vi "RT Loop - Analyze Acceleration_3.vi"(7 "testing":bool, 8 "error in (no error)":errorcluster, 9 "Acceleration RT FIFO In":T1, 10 "FPGA VI Reference Out":refnum<k20>, 11 "Message Queue":refnum<queue>) -> (1 "Acceleration RT FIFO Out":T1)   [LabVIEW 2017]
doc: "Read and analyze acceleration waveform data from FPGA via DMA FIFO. If the acceleration is over the limit, then send the acceleration waveform data to the Log Data Loop."
uses:
  UI Error Handlers/support/Message Queue/Message Cluster.ctl
  controls/Acceleration RT FIFO Reference.ctl
  Globals/Global - All RT Loop Stop.vi
  Globals/Global - Configuration Options.vi
  <vilib>/Utility/error.llb/Error Cluster From Error Code.vi
  <vilib>/rvi/errors/niLvFpgaAdjustHostInterfaceError.vi
  <vilib>/rvi/interface/nirviMethod/nirviMethod.xnode
  <vilib>/FPGAPlugInAG/Dynamic/niLvFpga_ReadFifo_Dynamic.vi
  <vilib>/rvi/errors/niLvFpgaMergeErrorWithErrorCode.vi
  UI Error Handlers/support/Logging/Logging.lvlib
  UI Error Handlers/support/Message Queue/Message Queue.lvlib
panel:
  out "Array":waveform(dbl)[](array[waveform])
  out "x-y":u32
  out "G1 status.G1 trigger":bool
  out "sta":bool
  out "logical OR":bool
  in  "Data Rate (Hz)":dbl
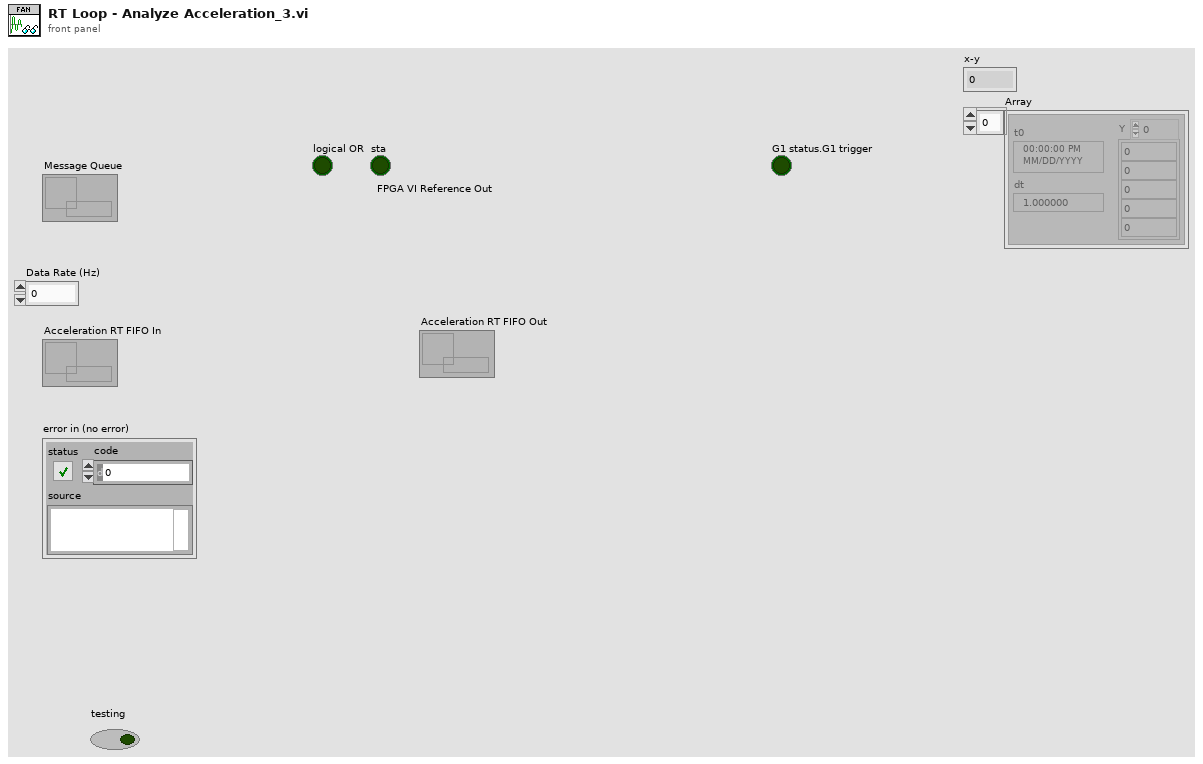
[diagram p1: front panel]
types:
  T1 = typedef "Acceleration RT FIFO Reference.ctl" = refnum<k33>
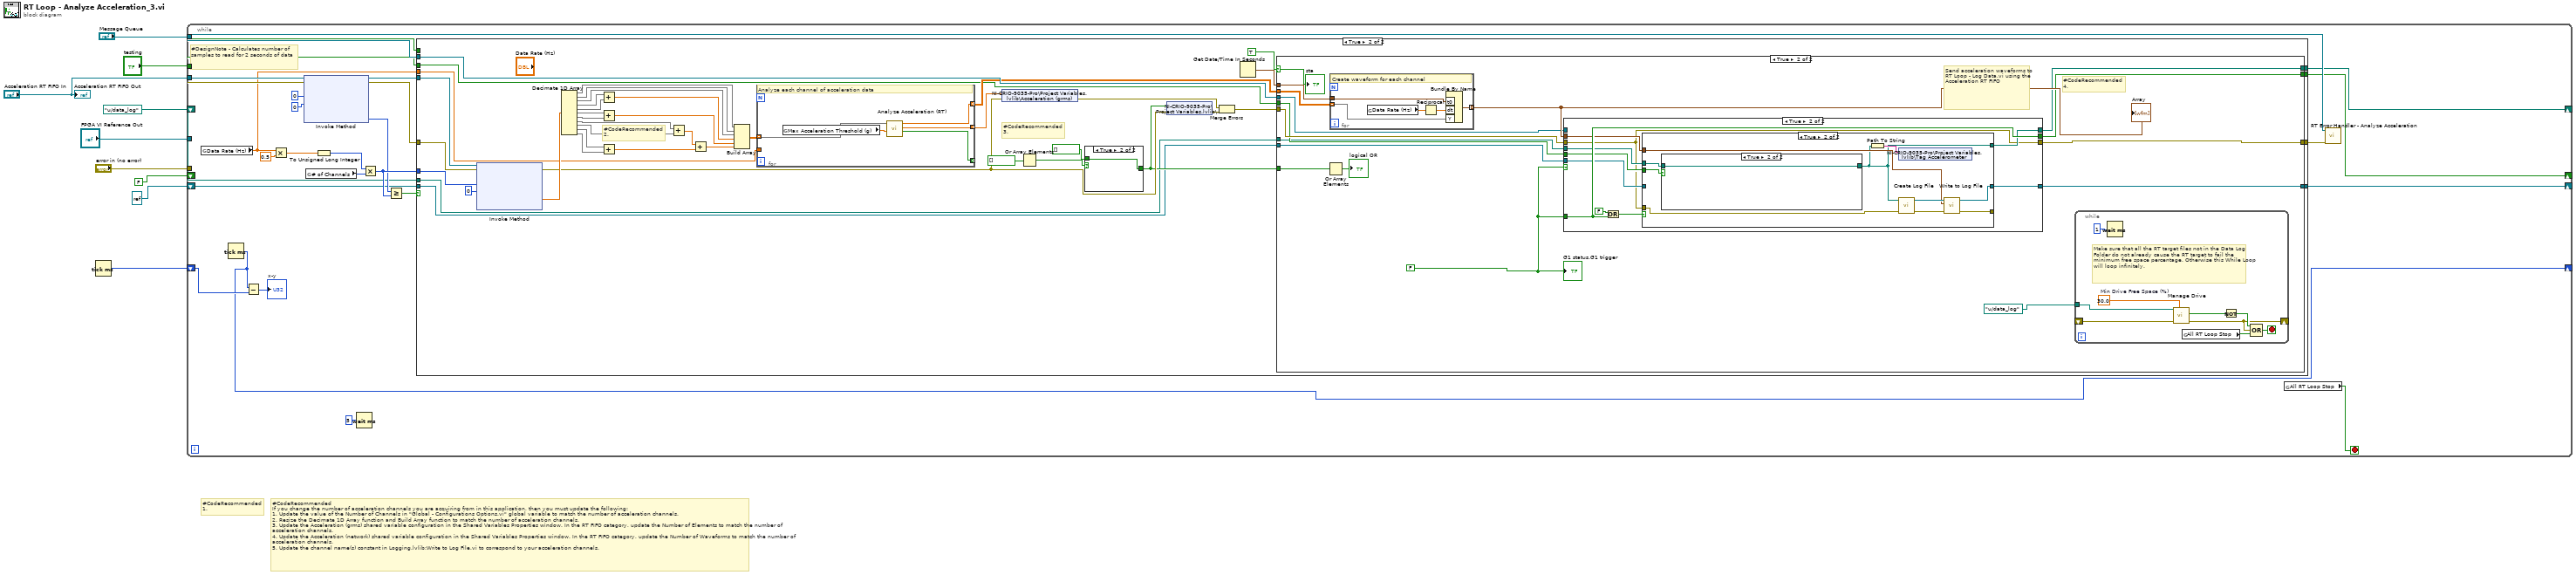
[diagram p0: block diagram]
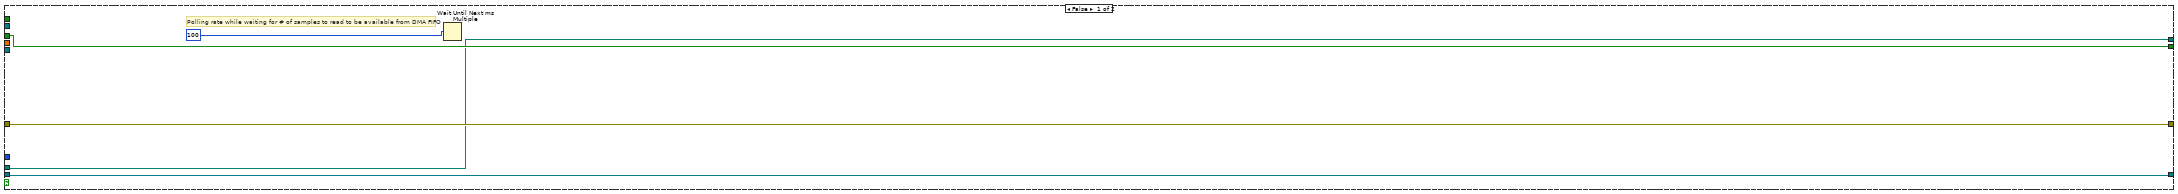
[diagram p2: hidden frame]
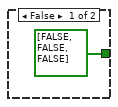
[diagram p3: hidden frame]
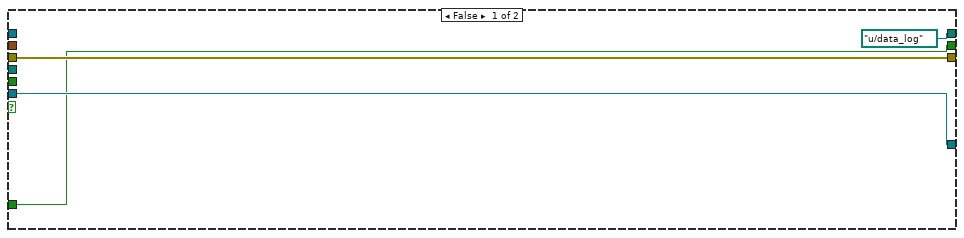
[diagram p5: hidden frame]
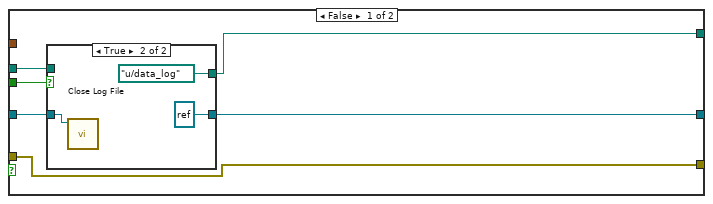
[diagram p6: hidden frame]
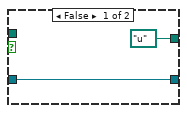
[diagram p7: hidden frame]
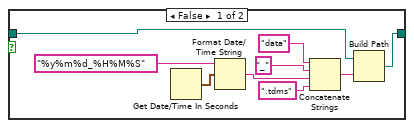
[diagram p8: hidden frame]
diagram:
  # "#CodeRecommended\n1."
  # "#CodeRecommended\nIf you change the number of acceleration channels you are acquiring from in this application, then you must update the following:\n1. Update the value of the Number of Channels in \"Global - Configurations Options.vi\" global variable to match the number of acceleration channels.\n2. Resize the Decimate 1D Array function and Build Array function to match the number of acceleration channels. \n3. Update the Acceleration (grms) shared variable configuration in the Shared Variables Properties window. In the RT FIFO category, update the Number of Elements to match the number of acceleration channels. \n4. Update the Acceleration (network) shared variable configuration in the Shared Variables Properties window. In the RT FIFO category, update the Number of Waveforms to match the number of acceleration channels.\n5. Update the channel name(s) constant in Logging.lvlib:Write to Log File.vi to correspond to your acceleration channels."
  n1 = Tick Count (ms)() -> (millisecond timer value=w1:u32)
  n2 = while {
    tunnel: "FPGA VI Reference Out" -> [w38]
    tunnel: "error in (no error)" -> [w37]
    tunnel: "Message Queue" -> [w30]
    tunnel: "Acceleration RT FIFO In" -> [w28]
    tunnel: "testing" -> [w20]
    shift-right: [w17] -> _
    shift-left: path "u:/data_log" ("AVI Path") -> [w16]
    shift-right: [w19] -> _
    shift-left: FALSE -> [w18]
    shift-right: [w15] -> _
    shift-left: refnum<k34> refnum ("Log File out") -> [w14]
    shift-right: [w12] -> _
    shift-left: w1 -> [w13]
    stop <- w31 stop-if-true
    # "#DesignNote - Calculates number of samples to read for 2 seconds of data"
    n3 = global read "Global - Configuration Options.vi" "Data Rate (Hz)"() -> (w22:dbl)
    n4 = Tick Count (ms)() -> (millisecond timer value=w12:u32)
    n5 = Subtract(x=w12, y=w13) -> (x-y=→"x-y":u32)
    n6 = Multiply(x=w22, y=0.5) -> (x*y=w26:dbl)
    n7 = xnode "Invoke Method"("FPGA VI Reference In"=w38, "error in"=w37, "Number of Elements"=u32 0, "Timeout (ms)"=0) -> ("FPGA VI Reference Out"=w34:refnum<k20>, "error out"=w33:errorcluster, "Elements Remaining"=w21:u32)  [unwired: 1 out]
    n8 = global read "Global - Configuration Options.vi" "# of Channels"() -> (w23:u32)
    n9 = To Unsigned Long Integer(number=w26) -> (unsigned 32bit integer=w25:u32)
    n10 = Wait (ms)(milliseconds to wait=u32 5) -> ()  [unwired: 1 out]
    n11 = Multiply(x=w25, y=w23) -> (x*y=w24:u32)
    n12 = Greater Or Equal?(x=w21, y=w24) -> (x >= y?=w32:bool)
    n13 = case shown="True" w32 {
      tunnel: w34 -> [_ w86]
      tunnel: w33 -> [w43 w85]
      tunnel: [w43 w81] -> w29
      tunnel: w24 -> [_ w84]
      tunnel: w28 -> [_ w80]
      tunnel: w22 -> [_ w76]
      tunnel: w20 -> [_ _]
      tunnel: [w41 w69] -> w19
      tunnel: w18 -> [w41 w68]
      tunnel: [w40 w67] -> w17
      tunnel: w16 -> [w40 w66]
      tunnel: [w39 w65] -> w15
      tunnel: w14 -> [w39 w64]
      frame False {
        # "Polling rate while waiting for # of samples to read to be available from DMA FIFO"
        n14 = Wait Until Next ms Multiple(millisecond multiple=u32 100) -> ()  [unwired: 1 out]
      }
      frame True {
        # "#CodeRecommended\n3."
        # "#CodeRecommended\n2."
        n15 = xnode "Invoke Method"("FPGA VI Reference In"=w86, "error in"=w85, "Number of Elements"=w84, "Timeout (ms)"=0) -> ("error out"=w75:errorcluster, "Data"=w79:sgl[])  [unwired: 2 out]
        n16 = Decimate 1D Array(w79) -> (w61:sgl[], w60:sgl[], w59:sgl[], w58:sgl[], w57:sgl[], w55:sgl[], w54:sgl[], w53:sgl[], w52:sgl[], w51:sgl[], w50:sgl[])
        n17 = Add(x=w58, y=w57) -> (x+y=w56:sgl[])
        n18 = Add(x=w55, y=w54) -> (x+y=w46:sgl[])
        n19 = Add(x=w51, y=w50) -> (x+y=w48:sgl[])
        n20 = Add(x=w53, y=w52) -> (x+y=w49:sgl[])
        n21 = Add(x=w49, y=w48) -> (x+y=w47:sgl[])
        n22 = Build Array(w61, w60, w59, w56, w46, w47) -> (w62:sgl[][])
        n23 = for {
          tunnel: [w93] -> _ mode=indexing
          tunnel: [w92] -> w78 mode=indexing
          tunnel: [w91] -> w77 mode=indexing
          tunnel: w76 -> [_]
          tunnel: w62 -> [w89] mode=indexing
          # "Analyze each channel of acceleration data"
          n24 = global read "Global - Configuration Options.vi" "Max Acceleration Threshold (g)"() -> (w90:sgl)
          n25 = call "Analyze Acceleration (RT).vi"("Max Instantaneous Acceleration (g)"=w90, "Acceleration Waveform (SGL)"=w89) -> ("Over Limit?"=w93:bool, "Acceleration (grms)"=w91:dbl, "Acceleration Waveform (DBL)"=w92:dbl[])  [unwired: 7 in]
        }
        n26 = shared-variable "NI-CRIO-9035-Pro\\Project Variables.lvlib\\Acceleration (grms)"(w77, error in=w75) -> (error out=w73:errorcluster)
        n27 = Or Array Elements(Boolean array=bool[] []) -> (logical OR=w71:bool)
        n28 = case shown="True" w71 {
          tunnel: bool[] [] -> [_ w88]
          tunnel: [bool[] [FALSE, FALSE, FALSE] ("Chatter?") w88] -> w70
          frame False {
          }
          frame True {
          }
        }
        n29 = shared-variable "NI-CRIO-9035-Pro\\Project Variables.lvlib\\Chatter?"(w70, error in=w75) -> (error out=w74:errorcluster)
        n30 = Merge Errors(w73, w74) -> (w72:errorcluster)
        n31 = Get Date/Time In Seconds() -> (seconds since 1Jan1904=w82:timestamp)
        n32 = case shown="True" TRUE {
          selector: TRUE -> [_ w107]
          tunnel: w82 -> [_ w114]
          tunnel: w72 -> [w97 w113]
          tunnel: [w97 w98] -> w81
          tunnel: w80 -> [_ w111]
          tunnel: w78 -> [_ w110]
          tunnel: w70 -> [_ w108]
          tunnel: [w96 w106] -> w69
          tunnel: w68 -> [w96 w105]
          tunnel: [w95 w104] -> w67
          tunnel: w66 -> [w95 w101]
          tunnel: [w94 w103] -> w65
          tunnel: w64 -> [w94 w102]
          frame False {
          }
          frame True {
            w99 = FALSE
            # "#CodeRecommended\n4."
            # "Send acceleration waveforms to RT Loop - Log Data.vi using the Acceleration RT FIFO"
            n33 = Or Array Elements(Boolean array=w108) -> (logical OR=→"logical OR":bool)
            n34 = for {
              tunnel: w110 -> [w173] mode=indexing
              tunnel: w114 -> [w172]
              tunnel: [w170] -> w112 mode=indexing
              # "Create waveform for each channel"
              n35 = global read "Global - Configuration Options.vi" "Data Rate (Hz)"() -> (w169:dbl)
              n36 = Reciprocal(x=w169) -> (1/x=w171:dbl)
              n37 = Bundle By Name("t0"=w172, "dt"=w171, "Y"=w173) -> (w170:waveform(dbl))  [unwired: 1 in]
            }
            "Array" <- w112
            n38 = case shown="True" w99 {
              tunnel: w113 -> [w127 w128]
              tunnel: w112 -> [_ w129]
              tunnel: w111 -> [_ _]
              tunnel: w99 -> [w125 w135]
              tunnel: [w125 w135] -> w106
              tunnel: w105 -> [_ w134]
              tunnel: [path "u:/data_log" ("AVI Path") w133] -> w104
              tunnel: w101 -> [_ w132]
              tunnel: [w126 w131] -> w103
              tunnel: w102 -> [w126 w130]
              tunnel: [w127 w128] -> w98
              frame False {
              }
              frame True {
                n39 = Or(x=FALSE, y=w135) -> (x .or. y?=w137:bool)
                n40 = case shown="True" w137 {
                  tunnel: w132 -> [w140 w158]
                  tunnel: [w143 w152] -> w133
                  tunnel: w134 -> [w141 w157]
                  tunnel: w130 -> [w142 _]
                  tunnel: w129 -> [_ w154]
                  tunnel: [w139 w151] -> w131
                  tunnel: w128 -> [w138 w150]
                  tunnel: [w138 w149] -> _
                  frame False {
                    n41 = case shown="True" w141 {
                      tunnel: [path "u:/" ("AVI Path") path "u:/data_log" ("AVI Path")] -> w143
                      tunnel: w142 -> [w144 w147]
                      tunnel: w140 -> [_ _]
                      tunnel: [w144 refnum<k34> refnum ("Log File out")] -> w139
                      frame False {
                      }
                      frame True {
                        n42 = call "Close Log File.vi"("tdms file"=w147) -> ()  [unwired: 10 in, 1 out]
                      }
                    }
                  }
                  frame True {
                    n43 = case shown="True" w157 {
                      tunnel: w158 -> [w160 w168]
                      tunnel: [w159 w168] -> w152
                      frame False {
                        n44 = Get Date/Time In Seconds() -> (seconds since 1Jan1904=w163:timestamp)
                        n45 = Format Date/Time String(time format string (%c)="%y%m%d_%H%M%S", seconds (now)=w163) -> (date/time string=w166:string)  [unwired: 1 out]
                        n46 = Concatenate Strings("data" ("string"), "_" ("string"), w166, ".tdms" ("string")) -> (w161:string)
                        n47 = Build Path(base path=w160, name or relative path=w161) -> (appended path=w159:path)
                      }
                      frame True {
                      }
                    }
                    n48 = Path To String(path=w152) -> (string=w153:string)
                    n49 = shared-variable "NI-CRIO-9035-Pro\\Project Variables.lvlib\\Tag Accelerometer"(w153) -> ()  [unwired: 1 in, 1 out]
                    n50 = call "Create Log File.vi"("error in (no error)"=w150, "Acceleration Exceeded Log Folder"=w152) -> ("error out"=w156:errorcluster, "Log File out"=w155:refnum<k34>)  [unwired: 8 in]
                    n51 = call "Write to Log File.vi"("error in (no error)"=w156, "Array of Waveforms"=w154, "Log File in"=w155) -> ("error out"=w149:errorcluster, "Log File out"=w151:refnum<k34>)  [unwired: 7 in]
                  }
                }
              }
            }
            n52 = while {
              shift-right: [w118] -> _
              shift-left: _ -> [w119]
              tunnel: path "u:/data_log" ("AVI Path") -> [w116]
              stop <- w123 stop-if-true
              w117 = 30.0  # Min Drive Free Space (%)
              # "Make sure that all the RT target files not in the Data Log Folder do not already cause the RT target to fail the minimum free space percentage. Otherwise this While Loop will loop infinitely."
              n53 = Wait (ms)(milliseconds to wait=u32 1) -> ()  [unwired: 1 out]
              n54 = call "Manage Drive.vi"("Min Drive Free Space (%)"=w117, "error in"=w119, "Data Folder"=w116) -> ("error out"=w118:errorcluster, "Drive Space Below Limit"=w115:bool)  [unwired: 7 in]
              n55 = global read "Global - All RT Loop Stop.vi" "All RT Loop Stop"() -> (w120:bool)
              n56 = Not(x=w115) -> (.not. x?=w122:bool)
              n57 = Compound Arithmetic op=OR(w122, w118, w120) -> (w123:bool)
            }
            "sta" <- w107
            "G1 status.G1 trigger" <- w99
          }
        }
      }
    }
    n58 = global read "Global - All RT Loop Stop.vi" "All RT Loop Stop"() -> (w31:bool)
    n59 = call "RT Error Handler - Analyze Acceleration.vi"("error in (no error)"=w29, "Message Queue"=w30) -> ()  [unwired: 9 in, 1 out]
  }
  "Acceleration RT FIFO Out" <- "Acceleration RT FIFO In"
